vi "单个流程写入.vi"(5 "简易流程Id":u16(ring), 6 "是否是简易流程":bool, 7 "添加的路径":path, 8 "error in (no error)":errorcluster caption="错误输入（无错误）", 9 "量程":enum16{"低量程", "高量程"}(ring), 10 "测量模式":T1(ring), 11 "测量参数":u16(ring) items=["总氮"=2, "总磷"=1, "氨氮"=3, "COD"=22]) -> (0 "error out":errorcluster caption="错误输出", 3 "步数":i32)   [LabVIEW 2016, in "斯坦道总氮.lvlib"]
panel:
  out "流程写入进度":dbl
  out "数组 2":u16[][](array[numeric]) format="0x%04x"
  out "大小":i32
  out "交织的数组":u16[](array[numeric]) format="0x%04x"
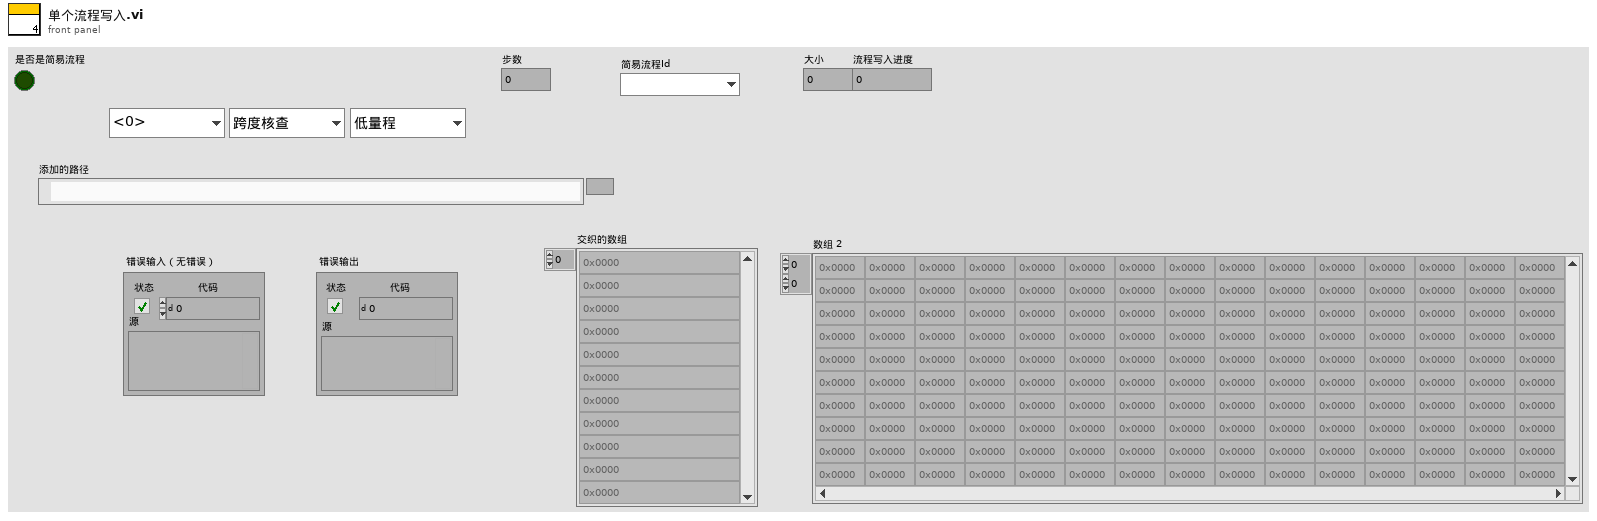
[diagram p1: front panel]
types:
  T1 = enum16{"跨度核查", "水样测量", "零点核查", "标样核查", "加标回收", "快捷测试", "空白校准", "标样校准"}
  T2 = cluster{"测量参数":u16, "测量模式":enum16{"跨度核查", "水样测量", "零点核查", "标样核查", "加标回收", "快捷测试", "空白校准", "标样校准"}, "量程":enum16{"低量程", "高量程"}}
  T3 = cluster{"port":u32, "dac":u8, "adc":u8, "time":u16, "步骤名":string}[]
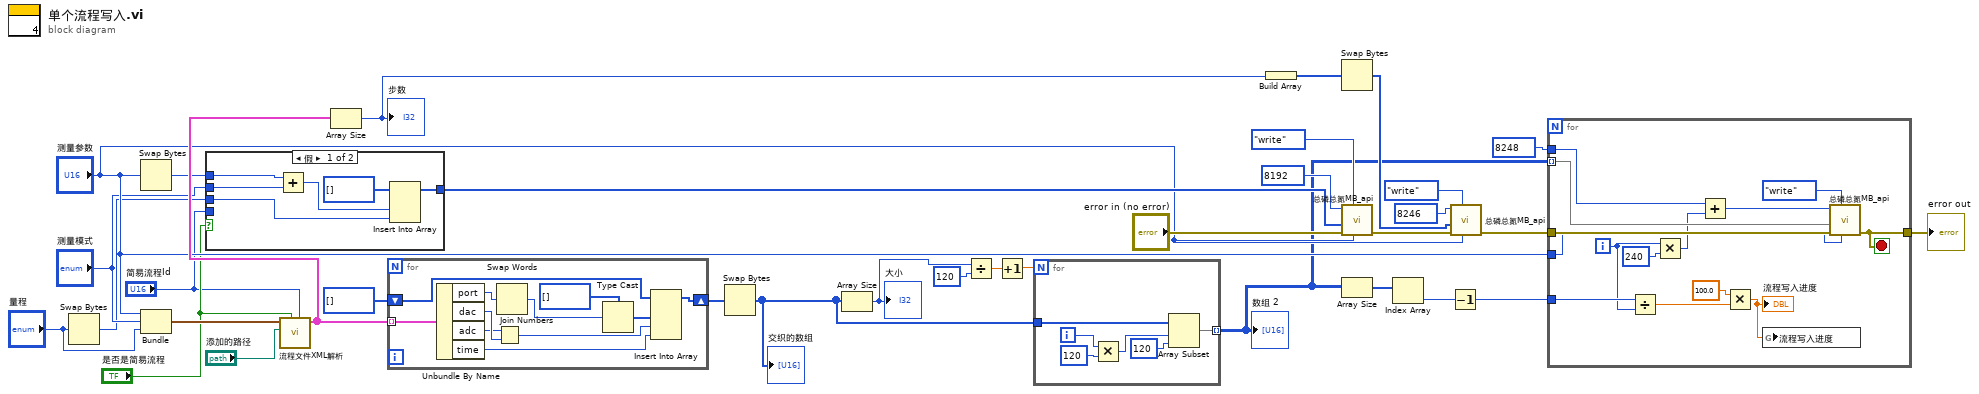
[diagram p0: block diagram]
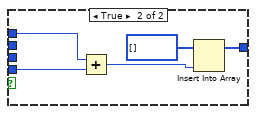
[diagram p2: hidden frame]
diagram:
  n1 = Swap Bytes(anything="量程") -> (byte swapped=w2:u16)
  n2 = Swap Bytes(anything="测量参数") -> (byte swapped=w12:u16)
  n3 = Bundle("测量参数"="测量参数", "测量模式"="测量模式", "量程"="量程") -> (w24:T2)  [unwired: 1 in]
  n4 = case shown="假" "是否是简易流程" {
    tunnel: [w38 w43] -> w28
    tunnel: "测量模式" -> [w37 _]
    tunnel: w12 -> [w36 w42]
    tunnel: w2 -> [w35 _]
    tunnel: "简易流程Id" -> [_ w41]
    frame False {
      n5 = Add(x=w36, y=w37) -> (x+y=w40:u16)
      n6 = Insert Into Array(array=u16[] [] ("数组"), new element #1=w40, new element #2=w35) -> (w38:u16[])  [unwired: 1 in]
    }
    frame True {
      n7 = Add(x=w42, y=w41) -> (x+y=w45:u16)
      n8 = Insert Into Array(array=u16[] [] ("数组"), new element=w45) -> (w43:u16[])  [unwired: 1 in]
    }
  }
  n9 = call "流程文件XML解析.vi"("简易流程Id"="简易流程Id", "是否是简易流程"="是否是简易流程", "添加的路径"="添加的路径", "参数簇"=w24) -> ("数组"=w18:T3)  [unwired: 7 in]
  n10 = Array Size(array=w18) -> (size(s)=w13:i32)
  "步数" <- w13
  n11 = for {
    tunnel: w18 -> [w56] mode=indexing
    shift-right: [w51] -> w21
    shift-left: u16[] [] -> [w49]
    n12 = Unbundle By Name(w56) -> ("port"=w54:u32, "dac"=w47:u8, "adc"=w46:u8, "time"=w52:u16)
    n13 = Join Numbers(hi=w46, lo=w47) -> ((hi.lo)=w53:u16)
    n14 = Swap Words(1:w54) -> (0:w48:u32)
    n15 = Type Cast(type=u16[] [], x=w48) -> (*(type *) &x=w50:u16[])
    n16 = Insert Into Array(array=w49, new element #1=w50, new element #2=w53, new element #3=w52) -> (w51:u16[])  [unwired: 1 in]
  }
  n17 = Swap Bytes(anything=w21) -> (byte swapped=w3:u16[])
  "交织的数组" <- w3
  n18 = Array Size(array=w3) -> (size(s)=w20:i32)
  "大小" <- w20
  n19 = Divide(x=w20, y=120) -> (x/y=w16:dbl)
  n20 = Increment(x=w16) -> (x+1=w15:dbl)
  n21 = for {
    N: w15 -> [_]
    tunnel: w3 -> [w60]
    tunnel: [w57] -> w7 mode=indexing
    i -> [w62]
    n22 = Multiply(x=w62, y=120) -> (x*y=w59:i32)
    n23 = Array Subset(array=w60, index=w59, length=120 ("y")) -> (w57:u16[])
  }
  "数组 2" <- w7
  n24 = Build Array(w13) -> (w17:i32[])
  n25 = Swap Bytes(anything=w17) -> (byte swapped=w14:i32[])
  n26 = call "总磷总氮MB_api.vi"("Slave ID"="测量参数", "STEP"=enum16{"open", "read", "write", "close"}."write", "Error in"="error in (no error)", "values"=w28, "starting address"=u16 8192) -> ("error out"=w31:errorcluster)  [unwired: 4 in, 2 out]
  n27 = Array Size(array=w7) -> (size(s)=w6:i32[])
  n28 = Index Array(array=w6) -> (element=w5:i32)  [unwired: 1 in]
  n29 = Decrement(x=w5) -> (x-1=w4:i32)
  n30 = call "总磷总氮MB_api.vi"("Slave ID"="测量参数", "STEP"=enum16{"open", "read", "write", "close"}."write", "Error in"=w31, "values"=w14, "starting address"=u16 8246) -> ("error out"=w27:errorcluster)  [unwired: 4 in, 2 out]
  n31 = for {
    tunnel: u16 8248 ("starting address") -> [w70]
    tunnel: w27 -> [w76]
    tunnel: [w74] -> w25
    tunnel: "测量参数" -> [w73]
    tunnel: w7 -> [w72] mode=indexing
    tunnel: w4 -> [w67]
    i -> [w66]
    stop <- w74 stop-if-true
    n32 = Divide(x=w67, y=w66) -> (x/y=w65:dbl)
    n33 = Multiply(x=w66, y=240) -> (x*y=w69:i32)
    n34 = Add(x=w70, y=w69) -> (x+y=w71:i32)
    n35 = Multiply(x=100.0, y=w65) -> (x*y=w63:dbl)
    "流程写入进度" <- w63
    n36 = global write "VAR总磷总氮全局变量.vi" "流程写入进度"(w63) -> ()
    n37 = call "总磷总氮MB_api.vi"("Slave ID"=w73, "STEP"=enum16{"open", "read", "write", "close"}."write", "Error in"=w76, "values"=w72, "starting address"=w71) -> ("error out"=w74:errorcluster)  [unwired: 4 in, 2 out]
  }
  "error out" <- w25
